vi "Tx Streaming (Host).vi"() -> ()   [LabVIEW 2013]
doc: "This template is for the Simple NI-USRP Streaming design, a design that shows the basics of streaming data from an NI 294x/295x device. Refer to the block diagram for more information about how to use this template."
uses:
  <vilib>/userdefined/Silver/nirio_resource_slv.ctl
  SubVIs/Start Trigger.ctl
  <vilib>/Utility/error.llb/DialogType.ctl
  SubVIs/Configure Signal (Level).vi
  SubVIs/Write Tx Data (I16 multi).vi
panel:
  in  "reference frequency source":string(combo)="Internal" caption="Reference Frequency Source"
  in  "tx active antenna":string(combo)="TX1" caption="Tx Active Antenna"
  in  "tx channel":string(combo)="tx/RF 1" caption="Tx Channel"
  in  "number of samples is finite":bool
  in  "USRP RIO device":T1="RIO0" caption="USRP RIO Device"
  in  "lo frequency":dbl=-1.0 caption="LO Frequency" format="%#.3pHz"
  in  "frequency":dbl=2000000000.0 caption="Frequency" format="%#.3pHz"
  in  "start trigger":T2=enum."Immediate" caption="Start Trigger"
  in  "output power":dbl caption="Output Power" format="%#_gdBm"
  in  "sample rate":dbl=10000000.0 caption="Sample Rate" format="%#.3pS/s"
  in  "number of samples":u32=1000000 caption="Number of Samples"
  out "Output Waveform":waveform(dbl)[](graph)
  in  "tone frequency":dbl=100000.0 caption="Tone Frequency" format="%#.3pHz"
  out "Generating":bool
  in  "stop":bool
  # "Tx Streaming"
  # "This template is for the Simple NI-USRP Streaming design, a design that shows the basics of streaming data from an NI 294x/295x device. See the block diagram for more information on how to use this template."
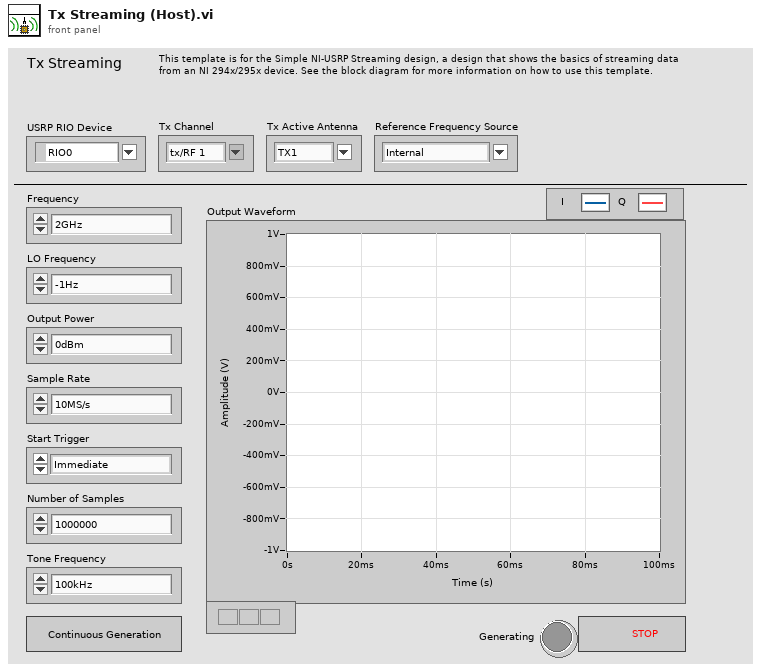
[diagram p1: front panel]
types:
  T1 = typedef "nirio_resource_slv.ctl" = tag
  T2 = typedef "Start Trigger.ctl" = enum8{"Software", "Digital Edge", "Rx Start Trigger", "Tx Start Trigger", "Immediate"}
  T3 = typedef "DialogType.ctl" = u16
  T4 = typedef "niUsrpRio Config v1 Host.lvlib/niUsrpRio Session.ctl" = cluster{"Global Settings Register Bus":T5, "Radio 0 Settings Register Bus":T5, "Rx NI-USRP session":refnum<k15>, "Tx NI-USRP session":refnum<k15>, "FPGA Interface":refnum<k20>, "RIO Interface Number":u32, "EEPROM Header":T6, "Device Data Header":T7, "EEPROM Characterization Header":T8, "Characterization Data":T9[], "Characterization Data Valid?":bool, "Radio 1 Settings Register Bus":T5, "Radio Settings Bus Semaphore":T11}
  T5 = typedef "niInstr Register Bus v0 Host.lvlib/Register Bus Session.ctl" = refnum<queue>
  T6 = typedef "niUsrpRio Config v1 Host.lvlib/EEPROM Header.ctl" = cluster{"Checksum":u32, "Product Code":u16, "Hardware Current Version":u16, "Hardware Oldest Compatible Version":u16, "EEPROM Map Current Version":u16, "EEPROM Map Oldest Compatible Version":u16, "User Password":string, "Pointer to Factory Header":u32, "Pointer to User Header":u32, "Recommended Interval":u16, "Number of Reserved Bytes":i32, "Number of Daughterboards":u8, "Daughterboard IDs":u16[], "Daughterboard Serial Numbers":string[]}
  T7 = typedef "niUsrpRio Config v1 Host.lvlib/EEPROM Device Data Header.ctl" = cluster{"Checksum":u32, "Number of Channels":u8, "Number of Gain Settings":u16[], "Pointer to Characterization Data":u32[], "Number of Reserved Bytes":i32, "Number of Frequencies":u16[]}
  T8 = typedef "niUsrpRio Config v1 Host.lvlib/EEPROM Characterization Header.ctl" = cluster{"Checksum":u32, "Date":timestamp, "Temperature":sgl, "Misc. Info":string, "Pointer to Device Data Header":u32, "Number of Reserved Bytes":i32}
  T9 = typedef "niUsrpRio Config v1 Host.lvlib/Characterization Data.ctl" = cluster{"Gains[dB]":dbl[], "Frequencies [Hz]":dbl[], "IQ Imbalance Table":T10[], "Measured Gains[dB]":dbl[][]}
  T10 = typedef "niUsrpRio Config v1 Host.lvlib/IQ Imbalance.ctl" = cluster{"Gain Imbalance [linear]":dbl, "Phase Imbalance [radians]":dbl, "Offset":cdb}
  T11 = typedef "Semaphore RefNum" = refnum<k1>
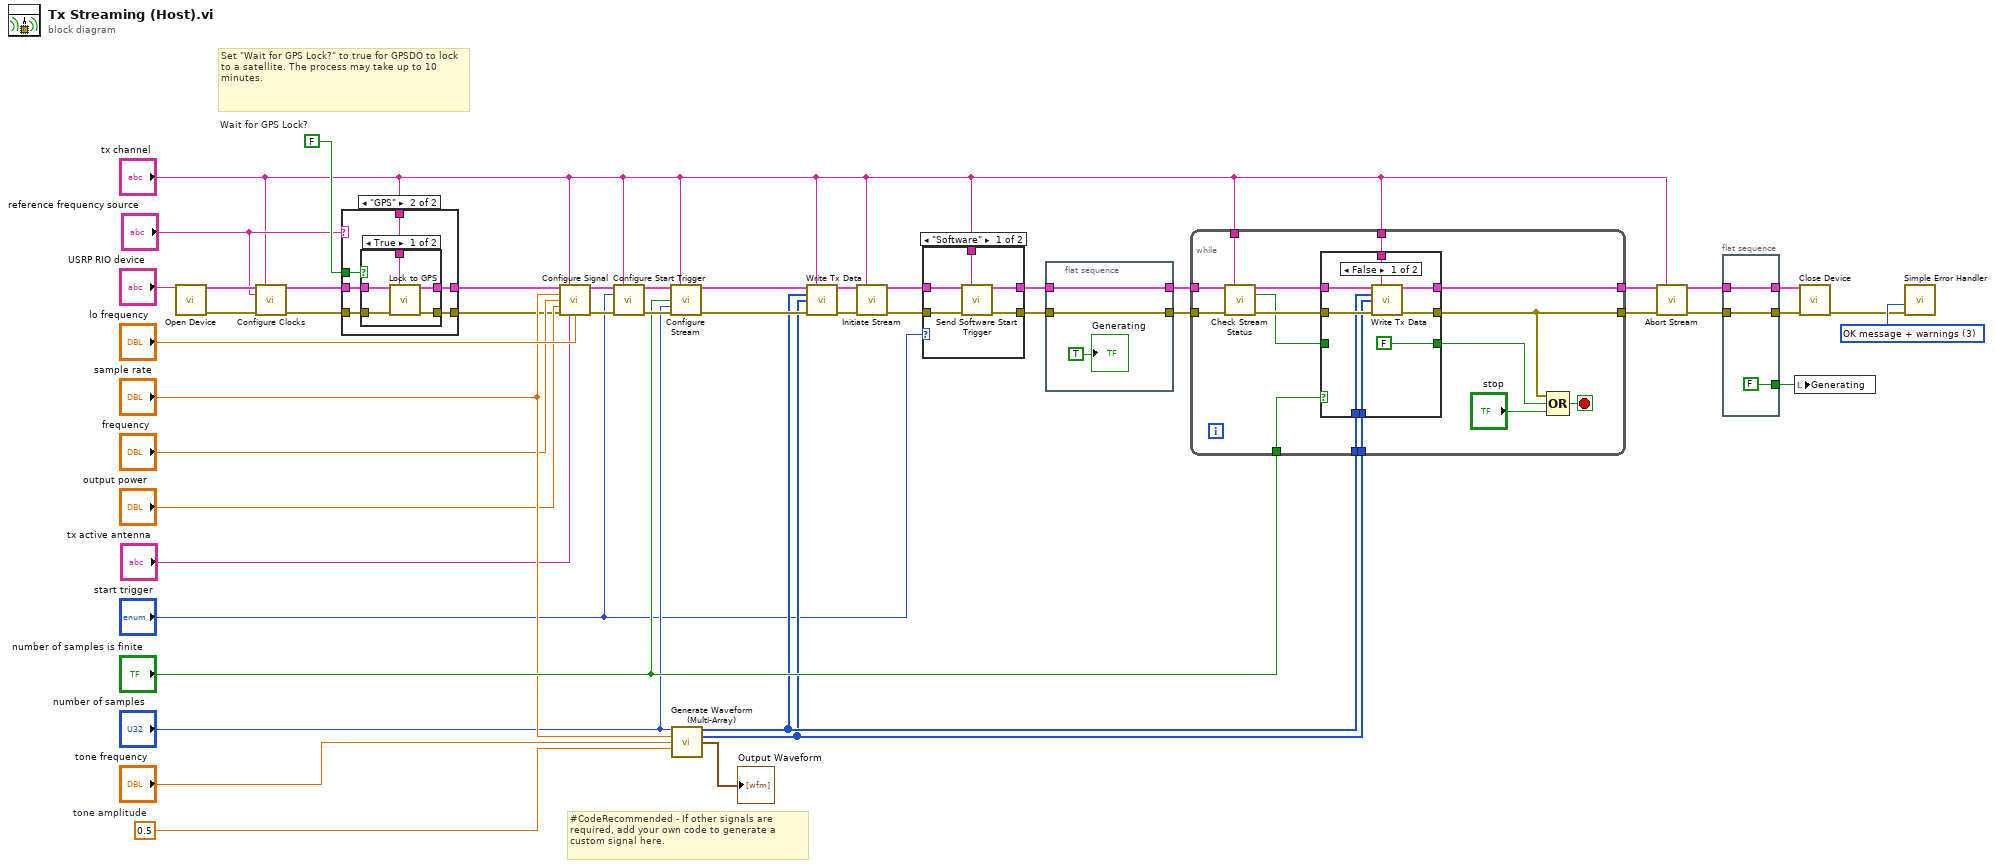
[diagram p0: block diagram]
diagram:
  w7 = FALSE  # Wait for GPS Lock?
  w15 = 0.5  # tone amplitude
  w39 = T3 3 items=["no dialog", "OK message", "continue or stop message", "OK message + warnings", "continue/stop + warnings"] ("type of dialog (OK msg:1)")
  # "Set \"Wait for GPS Lock?\" to true for GPSDO to lock to a satellite. The process may take up to 10 minutes."
  # "#CodeRecommended - If other signals are required, add your own code to generate a custom signal here."
  n1 = call "Open Device.vi"("USRP RIO device"="USRP RIO device") -> ("niUsrpRio Session (out)"=w30:T4, "error out"=w44:errorcluster)  [unwired: 13 in]
  n2 = call "Configure Clocks.vi"("niUsrpRio Session"=w30, "scope"="tx channel", "Reference Frequency Source"="reference frequency source", "error in"=w44) -> ("niUsrpRio Session (out)"=w5:T4, "error out"=w6:errorcluster)  [unwired: 10 in]
  n3 = case shown="\"GPS\"" "reference frequency source" {
    tunnel: w5 -> [w48 w54]
    tunnel: [w48 w53] -> w2
    tunnel: [w47 w52] -> w3
    tunnel: w6 -> [w47 w51]
    tunnel: "tx channel" -> [_ w50]
    tunnel: w7 -> [_ w49]
    frame Default {
    }
    frame "GPS" {
      n4 = case shown="True" w49 {
        tunnel: w54 -> [w56 w61]
        tunnel: [w59 w61] -> w53
        tunnel: [w58 w60] -> w52
        tunnel: w51 -> [w55 w60]
        tunnel: w50 -> [w57 _]
        frame True {
          n5 = call "Lock to GPS.vi"("niUsrpRio Session"=w56, "scope"=w57, "error in"=w55) -> ("niUsrpRio Session (out)"=w59:T4, "error out"=w58:errorcluster)  [unwired: 11 in]
        }
        frame False {
        }
      }
    }
  }
  n6 = call-poly "Configure Signal.vi"("niUsrpRio Session"=w2, "scope"="tx channel", "sample rate [S/s]"="sample rate", "frequency [Hz]"="frequency", "level [dBm]"="output power", "error in"=w3, "Active Antenna"="tx active antenna", "LO frequency [Hz]"="lo frequency") -> ("niUsrpRio Session (out)"=w31:T4, "error out"=w32:errorcluster)  [unwired: 1 in, 5 out]
  n7 = call "Configure Start Trigger.vi"("niUsrpRio Session"=w31, "scope"="tx channel", "start trigger"="start trigger", "error in"=w32) -> ("niUsrpRio Session (out)"=w29:T4, "error out"=w46:errorcluster)  [unwired: 10 in]
  n8 = call "Configure Stream.vi"("niUsrpRio Session"=w29, "scope"="tx channel", "number of samples is finite"="number of samples is finite", "number of samples"="number of samples", "error in"=w46) -> ("niUsrpRio Session (out)"=w27:T4, "error out"=w28:errorcluster)  [unwired: 9 in]
  n9 = call "Generate Waveform (Multi-Array).vi"("number of samples"="number of samples", "sample rate"="sample rate", "tone frequency"="tone frequency", "amplitude"=w15) -> ("I"=w23:i16[], "Q"=w22:i16[], "Waveform"=→"Output Waveform":waveform(dbl)[])  [unwired: 9 in]
  n10 = call-poly "Write Tx Data.vi"("niUsrpRio Session"=w27, "scope"="tx channel", "I"=w23, "Q"=w22, "error in"=w28) -> ("niUsrpRio Session (out)"=w37:T4, "error out"=w13:errorcluster)  [unwired: 9 in]
  n11 = call "Initiate Stream.vi"("niUsrpRio Session"=w37, "scope"="tx channel", "error in"=w13) -> ("niUsrpRio Session (out)"=w14:T4, "error out"=w18:errorcluster)  [unwired: 11 in]
  n12 = case shown="\"Software\"" "start trigger" {
    tunnel: w18 -> [w66 w68]
    tunnel: w14 -> [w64 w67]
    tunnel: [w65 w68] -> w12
    tunnel: [w63 w67] -> w11
    tunnel: "tx channel" -> [w62 _]
    frame "Software" {
      # "Send the software trigger to the master device only.  The master will also trigger all slave devices."
      n13 = call "Send Software Start Trigger.vi"("niUsrpRio Session"=w64, "scope"=w62, "error in"=w66) -> ("niUsrpRio Session (out)"=w63:T4, "error out"=w65:errorcluster)  [unwired: 11 in]
    }
    frame Default {
    }
  }
  n14 = flat-sequence {
    tunnel: w11 -> [w70]
    tunnel: w12 -> [w69]
    tunnel: [w70] -> w9
    tunnel: [w69] -> w10
    frame #0 {
      "Generating" <- TRUE ("Generating")
    }
  }
  n15 = while {
    tunnel: [w79] -> w20
    tunnel: w9 -> [w78]
    tunnel: w23 -> [w82]
    tunnel: w22 -> [w83]
    tunnel: w10 -> [w77]
    tunnel: [w75] -> w19
    tunnel: "number of samples is finite" -> [w74]
    tunnel: "tx channel" -> [w81]
    tunnel: "tx channel" -> [w80]
    stop <- w85 stop-if-true
    n16 = call "Check Stream Status.vi"("niUsrpRio Session"=w78, "scope"=w80, "error in"=w77) -> ("niUsrpRio Session (out)"=w76:T4, "done"=w73:bool, "error out"=w86:errorcluster)  [unwired: 10 in]
    n17 = case shown="False" w74 {
      tunnel: w86 -> [w94 w97]
      tunnel: w83 -> [w93 _]
      tunnel: w82 -> [w92 _]
      tunnel: w81 -> [w91 _]
      tunnel: [w89 w97] -> w75
      tunnel: [w90 w96] -> w79
      tunnel: w76 -> [w88 w96]
      tunnel: w73 -> [_ w95]
      tunnel: [FALSE ("done") w95] -> w72
      frame False {
        n18 = call-poly "Write Tx Data.vi"("niUsrpRio Session"=w88, "scope"=w91, "I"=w92, "Q"=w93, "error in"=w94) -> ("niUsrpRio Session (out)"=w90:T4, "error out"=w89:errorcluster)  [unwired: 9 in]
      }
      frame True {
      }
    }
    n19 = Compound Arithmetic op=OR(w75, w72, "stop") -> (w85:bool)
  }
  n20 = call "Abort Stream.vi"("niUsrpRio Session"=w20, "scope"="tx channel", "error in"=w19) -> ("niUsrpRio Session (out)"=w43:T4, "error out"=w42:errorcluster)  [unwired: 11 in]
  n21 = flat-sequence {
    tunnel: [w100] -> w40
    tunnel: w43 -> [w100]
    tunnel: [w99] -> w41
    tunnel: w42 -> [w99]
    tunnel: [FALSE ("Generating")] -> w34
    frame #0 {
    }
  }
  n22 = local write "Generating"(w34) -> ()
  n23 = call "Close Device.vi"("niUsrpRio Session"=w40, "error in"=w41) -> ("error out"=w38:errorcluster)  [unwired: 13 in]
  n24 = call <vilib>:"Simple Error Handler.vi"("type of dialog (OK msg:1)"=w39, "error in (no error)"=w38) -> ()  [unwired: 3 in, 5 out]
